vi "DivFrame.vi"(8 "error in":errorcluster, 10 "encode_data":dbl[](array[numeric]), 11 "Path In":path) -> (0 "error out":errorcluster, 2 "FreData":dbl[][](array[numeric]), 3 "Path Out":path, 4 "paddingBits":dbl format="%#_13g")   [LabVIEW 2015]
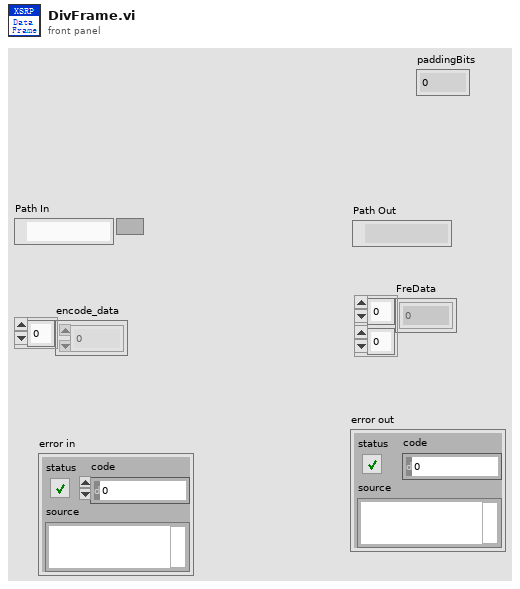
[diagram p1: front panel]
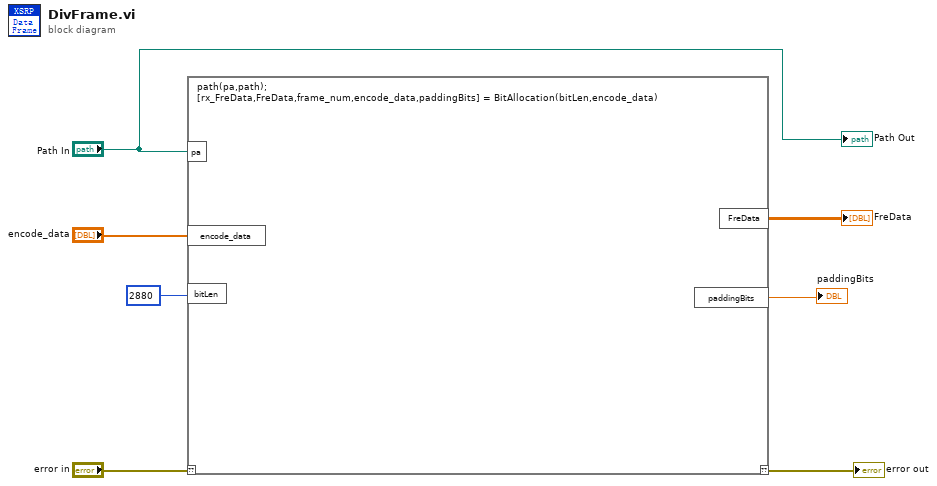
[diagram p0: block diagram]
diagram:
  n1 = script code="path(pa,path);\n[rx_FreData,FreData,frame_num,encode_data,paddingBits] = BitAllocation(bitLen,encode_data)"("??"="error in", "pa"="Path In", "encode_data"="encode_data", "bitLen"=2880) -> ("??"=→"error out":errorcluster, "FreData"=→"FreData":dbl[][], "paddingBits"=→"paddingBits":dbl)
  "Path Out" <- "Path In"
